vi "Test DataPoint.vi"() -> ()   [LabVIEW 2018, in "InfluxDB Client.lvlib"]
uses:
  Controls/FieldSet.ctl
  Controls/TagSet.ctl
  InfluxDB Client.lvlib
  Classes/DataPoint/DataPoint.lvclass
panel:
  out "Line protocol 1 tag 2 fields":string
  out "Line protocol 1 tag 1 field":string
  out "Line protocol 1 field":string
  out "Line protocol 2 tags 2 fields":string
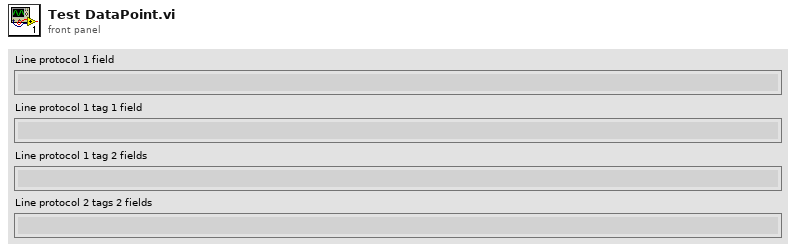
[diagram p1: front panel]
types:
  T1 = typedef "InfluxDB Client.lvlib/TagSet.ctl" = cluster{"Key":string, "Value":string}
  T2 = typedef "InfluxDB Client.lvlib/FieldSet.ctl" = cluster{"Key":string, "Value":variant}
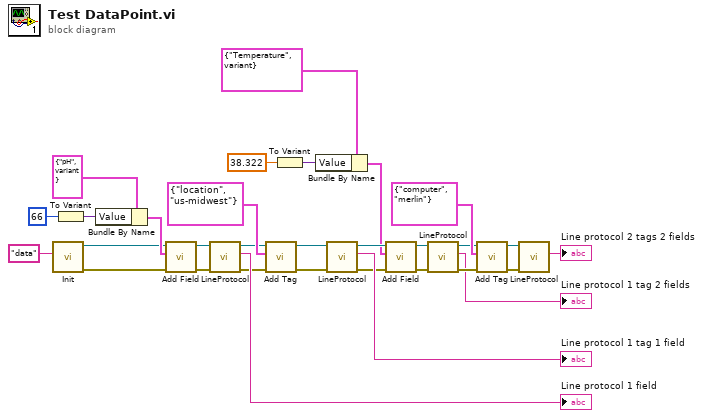
[diagram p0: block diagram]
diagram:
  n1 = call "Init.vi"("Measurement"="data") -> ("error out"=w1:errorcluster, "DataPoint out"=w2:refnum<class "DataPoint.lvclass">)  [unwired: 9 in]
  n2 = To Variant(anything=i8 66) -> (Variant=w25:variant)
  n3 = Bundle By Name(cluster=T2 {"Key"="pH", "Value"=variant} ("FieldSet"), "Value"=w25) -> (w24:T2)
  n4 = call "Add Field.vi"("error in (no error)"=w1, "FieldSet"=w24, "DataPoint in"=w2) -> ("error out"=w17:errorcluster, "DataPoint out"=w18:refnum<class "DataPoint.lvclass">)  [unwired: 7 in]
  n5 = call "LineProtocol.vi"("error in (no error)"=w17, "DataPoint in"=w18) -> ("error out"=w14:errorcluster, "Line protocol"=→"Line protocol 1 field":string, "DataPoint out"=w15:refnum<class "DataPoint.lvclass">)  [unwired: 7 in]
  n6 = call "Add Tag.vi"("error in (no error)"=w14, "TagSet"=T1 {"Key"="location", "Value"="us-midwest"}, "DataPoint in"=w15) -> ("error out"=w12:errorcluster, "DataPoint out"=w13:refnum<class "DataPoint.lvclass">)  [unwired: 7 in]
  n7 = To Variant(anything=38.322 ("temperature")) -> (Variant=w23:variant)
  n8 = Bundle By Name(cluster=T2 {"Key"="Temperature", "Value"=variant} ("FieldSet"), "Value"=w23) -> (w8:T2)
  n9 = call "LineProtocol.vi"("error in (no error)"=w12, "DataPoint in"=w13) -> ("error out"=w9:errorcluster, "Line protocol"=→"Line protocol 1 tag 1 field":string, "DataPoint out"=w10:refnum<class "DataPoint.lvclass">)  [unwired: 7 in]
  n10 = call "Add Field.vi"("error in (no error)"=w9, "FieldSet"=w8, "DataPoint in"=w10) -> ("error out"=w5:errorcluster, "DataPoint out"=w7:refnum<class "DataPoint.lvclass">)  [unwired: 7 in]
  n11 = call "LineProtocol.vi"("error in (no error)"=w5, "DataPoint in"=w7) -> ("error out"=w4:errorcluster, "Line protocol"=→"Line protocol 1 tag 2 fields":string, "DataPoint out"=w6:refnum<class "DataPoint.lvclass">)  [unwired: 7 in]
  n12 = call "Add Tag.vi"("error in (no error)"=w4, "TagSet"=T1 {"Key"="computer", "Value"="merlin"}, "DataPoint in"=w6) -> ("error out"=w28:errorcluster, "DataPoint out"=w29:refnum<class "DataPoint.lvclass">)  [unwired: 7 in]
  n13 = call "LineProtocol.vi"("error in (no error)"=w28, "DataPoint in"=w29) -> ("Line protocol"=→"Line protocol 2 tags 2 fields":string)  [unwired: 7 in, 2 out]
